vi "Trajectory Builder.vi"() -> ()   [LabVIEW 2018]
uses:
  <vilib>/event_ctls.llb/lveventtype.ctl
panel:
  in  "Time (s)":dbl(slide) scale=0.0..2.3600000000000003 scale format="%#.1g"
  in  "Play":bool
  in  "Destination":u16(ring) items=["Cargo", "Rocket"]
  in  "Direction":u16(ring) items=["Left", "Right", "Other"]
  out "fps":dbl[](graph)
  in  "Limits":T1={"Velocity (fps)"=6.0, "Acceleration (fps^2)"=15.0, "Jerk (fps^3)"=15.0} {"Jerk (fps^3)" min=0.0 step=10.0; "Acceleration (fps^2)" min=0.0; "Velocity (fps)" min=0.0}
  in  "Conditions":T2 {"vFinal (fps)" min=0.0; "vInitial (fps)" min=0.0}
  in  "Append":bool
  in  "Center Flip":bool
  out "WayPoints":cluster{"x":dbl, "y":dbl, "th":dbl}[](array[cluster]) {"th" format="%#_4g"}
  out "Distance (ft)":dbl format="%#.1g"
  in  "Open":i32(listbox)
  out "Path Status":bool
  in  "Sample Period (s)":dbl=0.02
  out "Duration (s)":dbl format="%#.1g"
  in  "Snap to foot":bool
  in  "Angle Limiter":enum16{"90", "45", "15", "1"}(ring)=enum."45"
  in  "Snap robot to baseline":bool
  in  "Filename":string
  in  "Save":bool
  in  "New":bool
  out "Picture":picture
  # "Directions:\nUse mouse to ...\n    move robot position (rectangle with arrow)\n    rotate robot (red arrow)\n    move waypoints (numbered circles)\nClick in open space to add a waypoint\nShift click to delete a waypoint\nHover over a waypoint and use arrow keys to nudge\n\nTime slider and Play button will run robot along path\nto test for collisions\n\nDirection and Destionation are folder selectors for files\n\nNew creates a new path at default location\n\nAppend creates a path"
  # "Trajectory Parameters"
  # "Interaction Options"
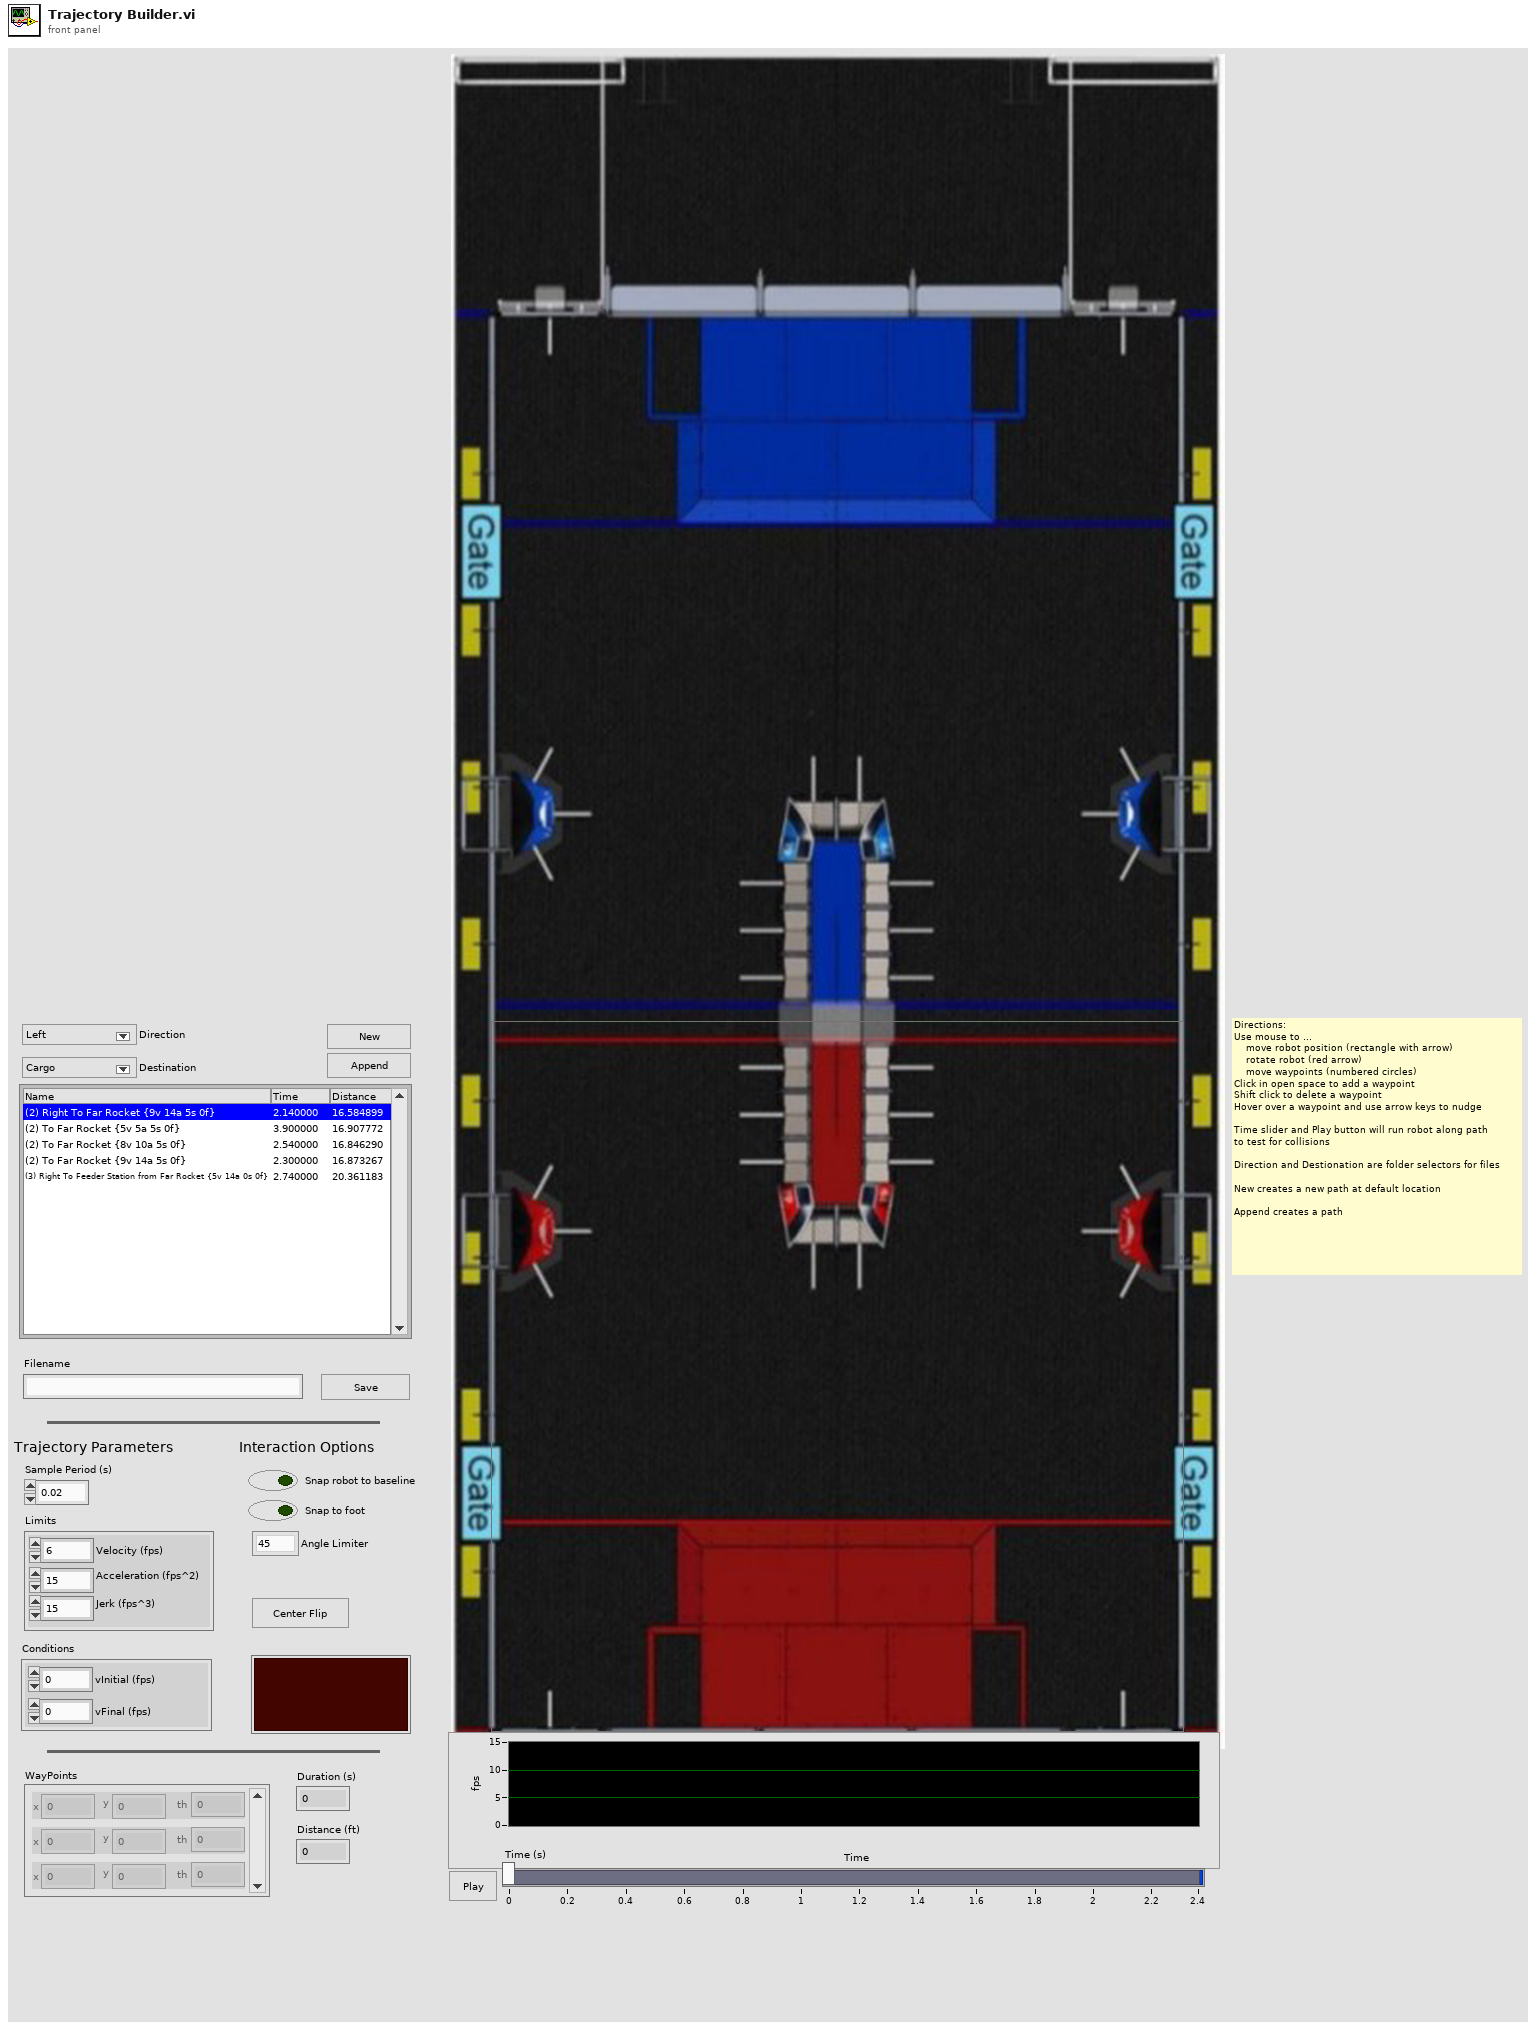
[diagram p1: front panel]
types:
  T1 = cluster{"Velocity (fps)":dbl, "Acceleration (fps^2)":dbl, "Jerk (fps^3)":dbl}
  T2 = cluster{"vInitial (fps)":dbl, "vFinal (fps)":dbl}
  T3 = cluster{"Name":string, "Color":u32, "Style":i32, "Point Style":i32, "Name Visible":bool, "Allow Drag":bool, "Annotation Mode":i32, "Plot":i32, "Index":i32, "Position":cluster{"X":dbl, "Y":dbl}, "X Scale":i32, "Y Scale":u32, "Show Arrow":bool, "Lock Name":bool, "Plot Area":i32, "Label Offset":cluster{"X":dbl, "Y":dbl}}
  T4 = cluster{"Index":i32, "Pt Test Results":enum16{"Miss", "Rect Hit", "Arrow Hit"}}
  T5 = enum16{"Accel Straight", "Const Straight", "Blend", "Circle"}
  T6 = cluster{"Velocity":dbl, "Sample Time":dbl, "Accel":dbl}
  T7 = cluster{"Segment Name":string, "Type":enum16{"Accel Straight", "Const Straight", "Blend", "Circle"}, "Traj Pos Points":cluster{"x":dbl, "y":dbl, "th":dbl}[], "Traj Vel Points":cluster{"V":dbl, "th":dbl}[], "Accel Index":i32, "Decel Index":i32}[]
  T8 = typedef "lveventtype.ctl" = enum32{"Null", "Timeout", "Annotation Menu Selection", "Annotation Menu Selection?", "App Instance Close", "App Instance Close?", "Autoscale Range Change", "Bookmark Info Change", "Cell Edit", "Cell Edit?", "Cursor Grab", "Cursor Grab?", "Cursor Menu Selection", "Cursor Menu Selection?", "Cursor Move", "Cursor Release", "Data Change", "Direction Change", "Display State Change", "Drag Ended", "Drag Enter", "Drag Leave", "Drag Over", "Drag Source Update", "Drag Starting", "Drag Starting?", "Drop", "Exec State Change", "Key Down", "Key Down?", "Key Repeat", "Key Repeat?", "Key Up", "Listbox Double Click", "Menu Activation?", "Menu Selection (App)", "Menu Selection? (App)", "Menu Selection (User)", "Mouse Down", "Mouse Down?", "Mouse Enter", "Mouse Leave", "Mouse Move", "Mouse Up", "Mouse Wheel", "NI Security User Change (App)", "Pane Size", "Panel Close", "Panel Close?", "Panel Resize", "Plot Attribute Change", "Scale Range Change", "Shortcut Menu Activation?", "Shortcut Menu Selection (App)", "Shortcut Menu Selection? (App)", "Shortcut Menu Selection (User)", "Tree Double Click", "Tree Drag", "Tree Drag?", "Tree Drop", "Tree Drop?", "Tree Item Close", "Tree Item Close?", "Tree Item Open", "Tree Item Open?", "User Event", "Value Change"}
  T9 = typedef "LVPoint32TypeDef.ctl" = cluster{"Horizontal":i32, "Vertical":i32}
  T10 = cluster{"Shift":bool, "Ctrl":bool, "Alt":bool, "Cmd":bool, "Opt":bool}
  T11 = typedef "LVPositionTypeDef.ctl" = cluster{"Left":i32, "Top":i32}
  T12 = typedef "LVBoundsTypeDef.ctl" = cluster{"Width":u32, "Height":u32}
  T13 = cluster{"Velocity":dbl, "Accel":dbl, "Accel":dbl}
  T14 = cluster{"Sample Period (s)":dbl, "Limits":cluster{"Velocity (fps)":dbl, "Acceleration (fps^2)":dbl, "Jerk (fps^3)":dbl}, "Conditions":cluster{"vInitial (fps)":dbl, "vFinal (fps)":dbl}}
  T15 = cluster{"Snap robot to baseline":bool, "Snap to foot":bool, "Angle Limiter":enum16{"90", "45", "15", "1"}}
  T16 = cluster{i32, "Pt Test Results":enum16{"Miss", "Rect Hit", "Arrow Hit"}}
  T17 = typedef "eventvkey.ctl" = enum16{"ASCII", "Enter", "Return", "Shift", "Ctrl", "Alt", "Cmd", "Opt", "Caps", "NumLock", "Clear", "Break", "Up", "Down", "Left", "Right", "Insert", "Delete", "Home", "End", "PageUp", "PageDown", "Escape", "Help", "Pause", "ScrollLock", "F1", "F2", "F3", "F4", "F5", "F6", "F7", "F8", "F9", "F10", "F11", "F12", "F13", "F14", "F15", "F16", "F17", "F18", "F19", "F20", "F21", "F22", "F23", "F24", "Play", "VolumeUp", "VolumeDown", "Mute", "Two Byte Char"}
  T18 = cluster{"Horizontal":dbl, "Vertical":dbl, "th":dbl}
  T19 = cluster{"Name":string, "Color":u32, "Style":i32, "Point Style":i32, "Name Visible":bool, "Allow Drag":bool, "Annotation Mode":i32, "Plot":i32, "Index":i32, "Position":cluster{"X":dbl, "Y":dbl}, "X Scale":i32, "Y Scale":u32, "Show Arrow":bool, "Lock Name":bool, "Plot Area":i32, "Label Offset":cluster{"X":dbl, "Y":dbl}}[]
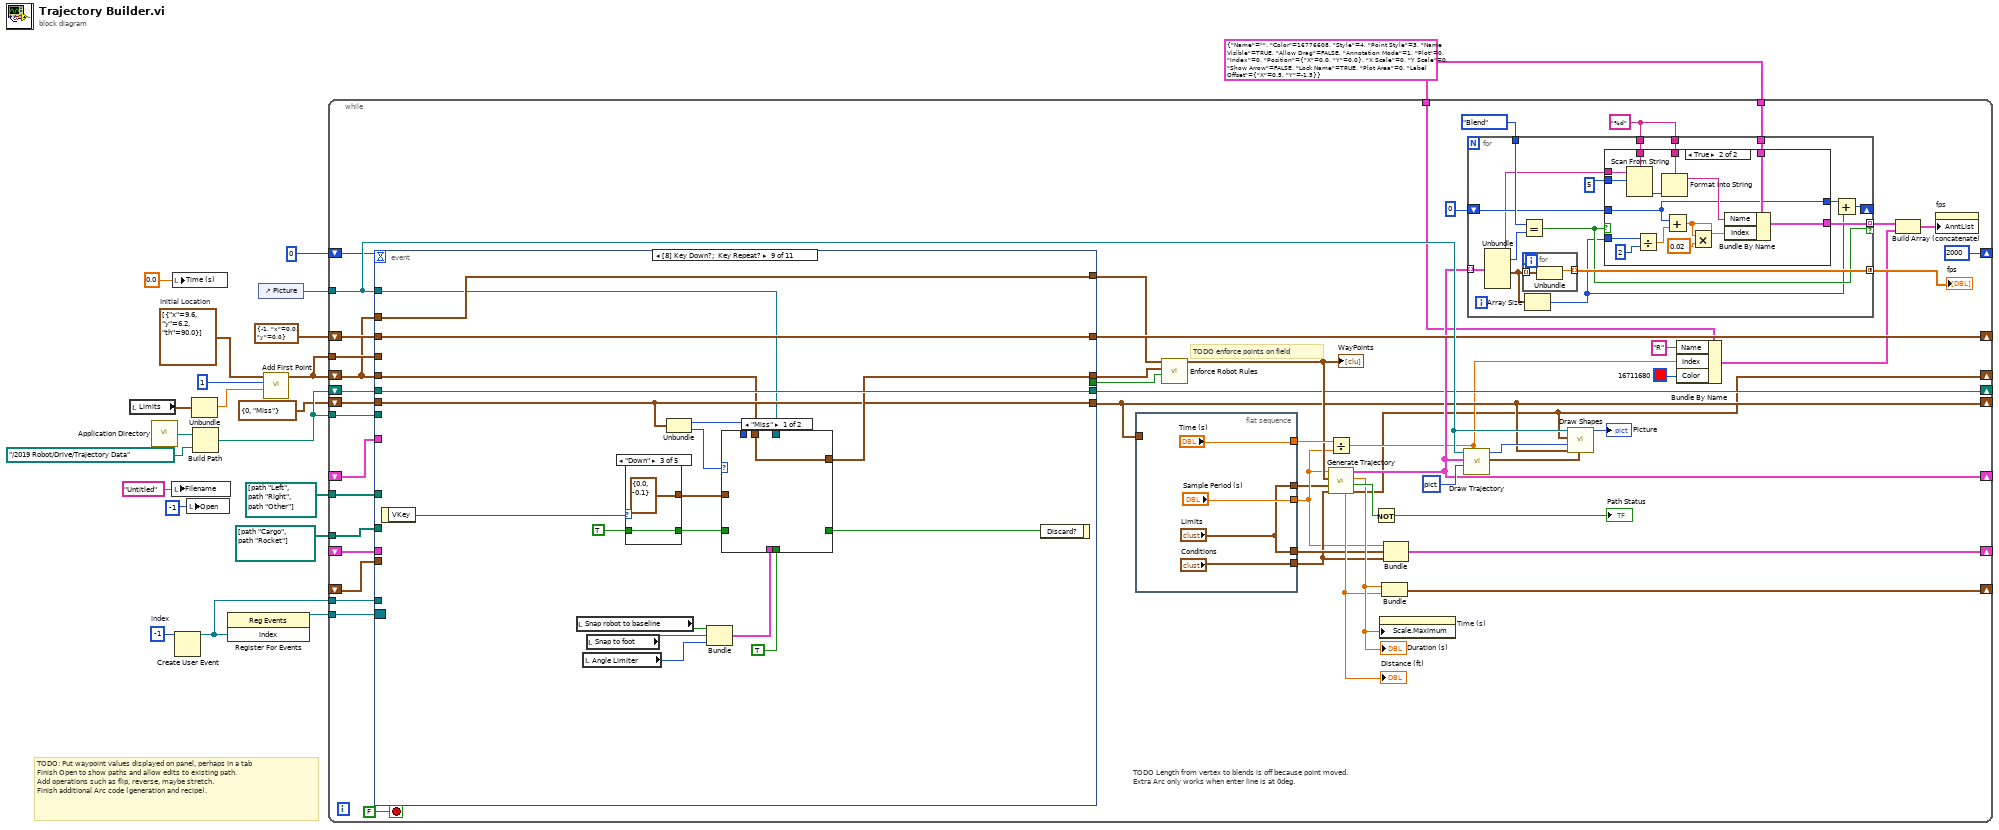
[diagram p0: block diagram]
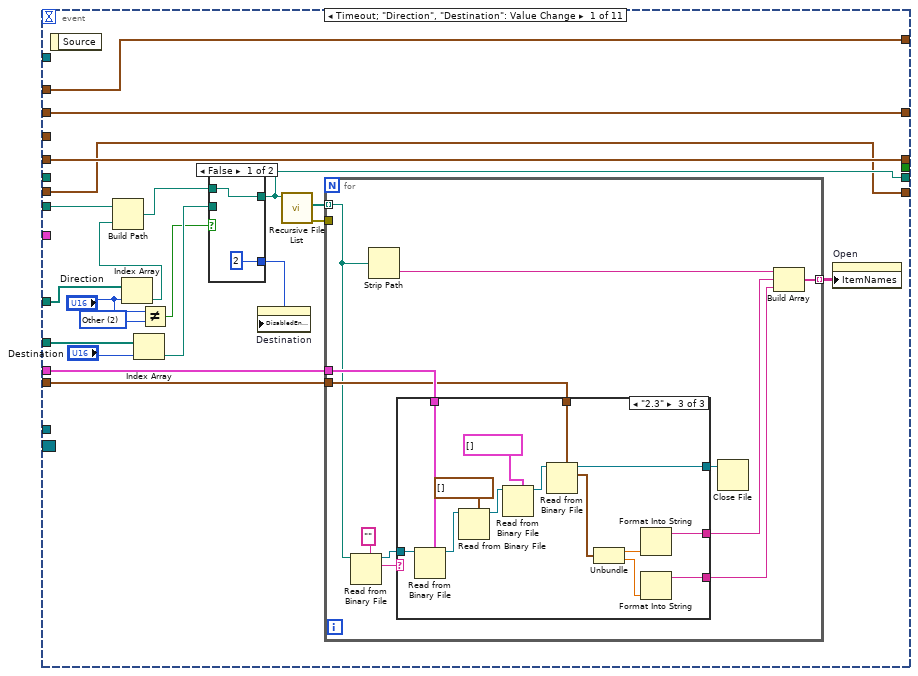
[diagram p3: hidden frame]
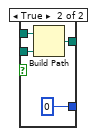
[diagram p4: hidden frame]
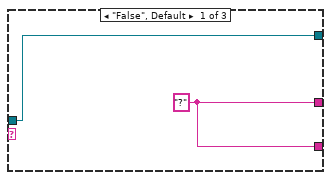
[diagram p5: hidden frame]
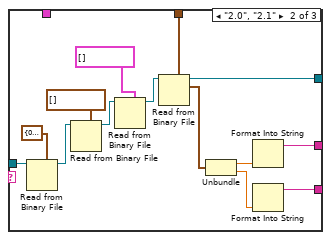
[diagram p6: hidden frame]
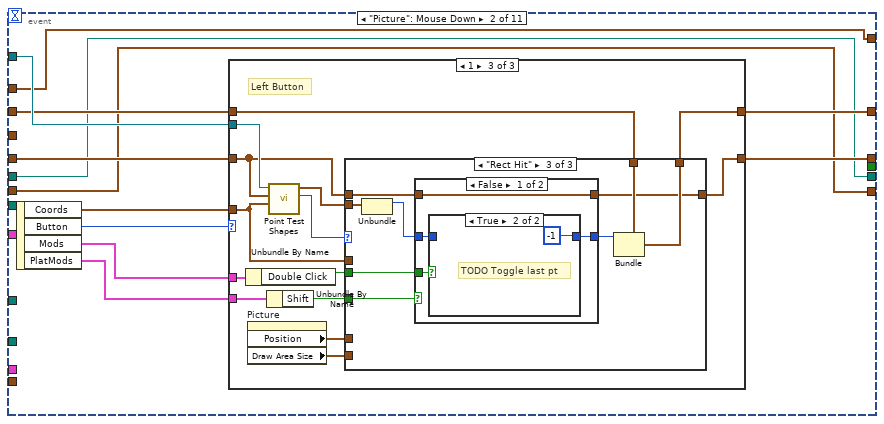
[diagram p7: hidden frame]
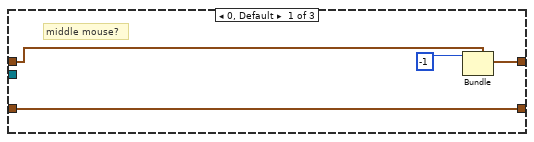
[diagram p8: hidden frame]
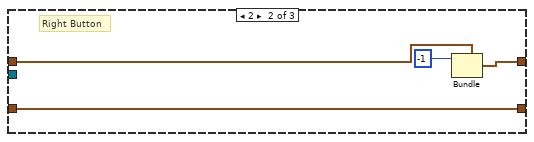
[diagram p9: hidden frame]
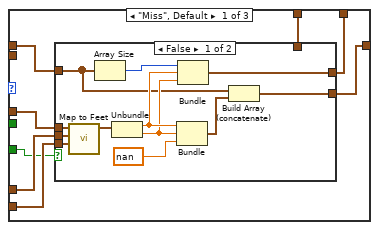
[diagram p10: hidden frame]
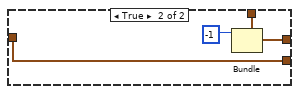
[diagram p11: hidden frame]
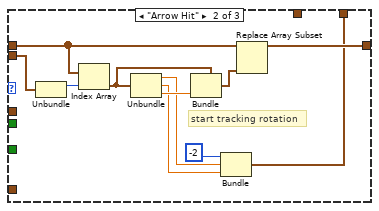
[diagram p12: hidden frame]
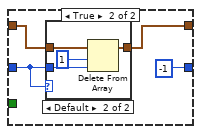
[diagram p14: hidden frame]
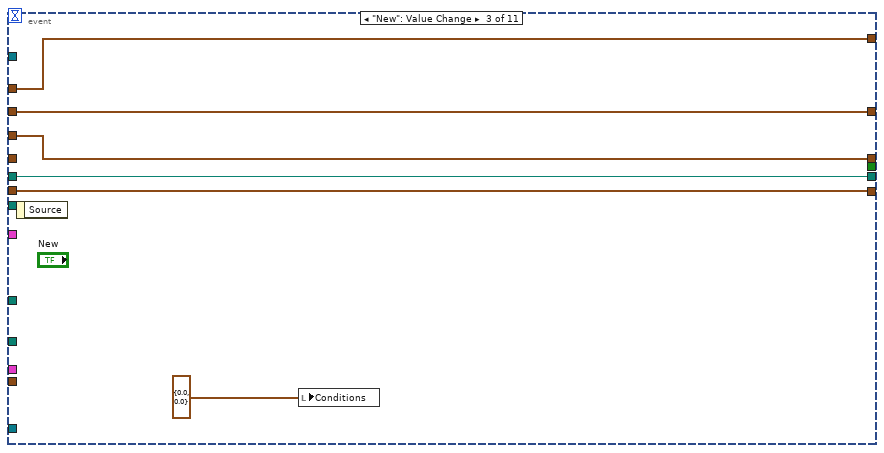
[diagram p16: hidden frame]
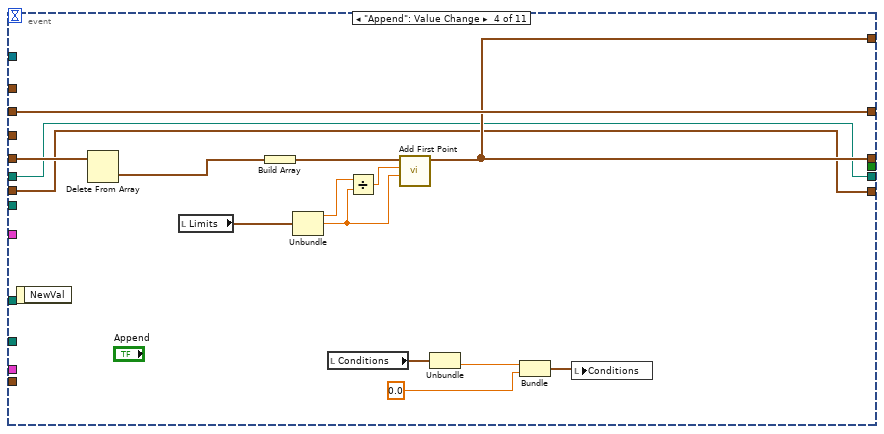
[diagram p17: hidden frame]
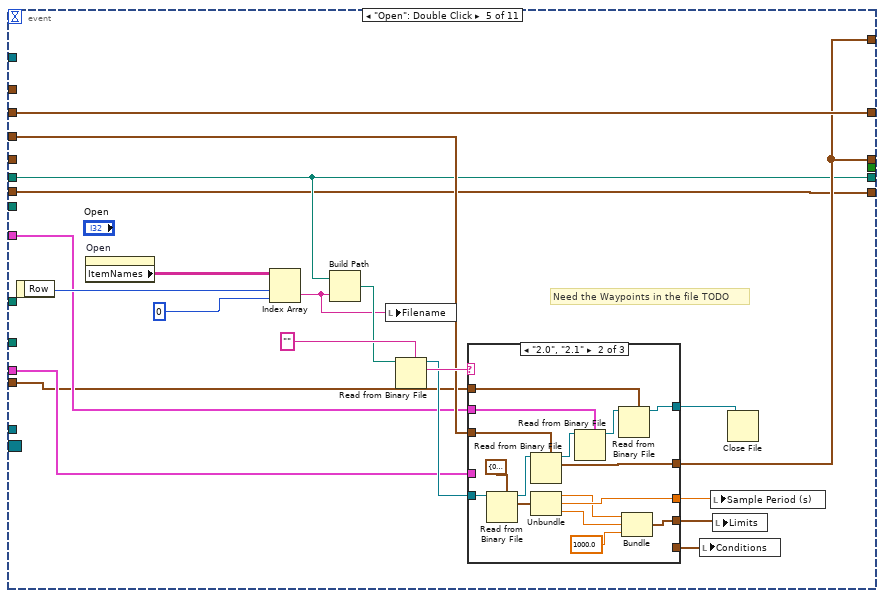
[diagram p18: hidden frame]
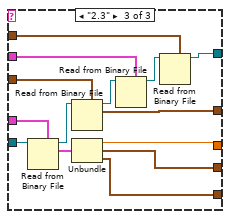
[diagram p20: hidden frame]
diagram:
  w1 = -1  # index
  w4 = T3 {"Name"="", "Color"=16776608, "Style"=4, "Point Style"=3, "Name Visible"=TRUE, "Allow Drag"=FALSE, "Annotation Mode"=1, "Plot"=0, "Index"=0, "Position"={"X"=0.0, "Y"=0.0}, "X Scale"=0, "Y Scale"=0, "Show Arrow"=FALSE, "Lock Name"=TRUE, "Plot Area"=0, "Label Offset"={"X"=0.5, "Y"=-1.5}}
  w18 = cluster{"x":dbl, "y":dbl, "th":dbl}[] [{"x"=9.6, "y"=6.2, "th"=90.0}]  # Initial Location
  # "TODO: Put waypoint values displayed on panel, perhaps in a tab\nFinish Open to show paths and allow edits to existing path.\nAdd operations such as flip, reverse, maybe stretch.\nFinish additional Arc code (generation and recipe)."
  n1 = local read "Limits"() -> (w12:T1)
  n2 = call <vilib>:"Application Directory.vi"() -> ("Application Directory"=w15:path)
  n3 = local write "Filename"("Untitled" ("Filename")) -> ()
  n4 = local write "Time (s)"(0.0 ("Time")) -> ()
  n5 = Create User Event(user event datatype=w1) -> (user event=w2:refnum<user-event>)  [unwired: 1 in, 1 out]
  n6 = local write "Open"(-1) -> ()
  n7 = Unbundle(w12) -> ("Acceleration (fps^2)"=w11:dbl)  [unwired: 2 out]
  n8 = Build Path(base path=w15, name or relative path=path "../2019 Robot/Drive/Trajectory Data") -> (appended path=w8:path)
  n9 = register-events(w2) -> (reference out=w3:refnum<event-registration>)  [unwired: 2 in, 1 out]
  n10 = control-ref of="Picture"() -> (w21:refnum<vi>)
  n11 = call "Add First Point.vi"("Accel (f/s^2)"=w11, "Time (s)"=1 ("th"), "Initial Points"=w18) -> ("Points"=w17:cluster{"x":dbl, "y":dbl, "th":dbl}[])  [unwired: 8 in]
  n12 = while {
    shift-right: [w24] -> _
    shift-left: w17 -> [w60]
    tunnel: w17 -> [w73]
    tunnel: w21 -> [w71]
    shift-right: [w53] -> _
    shift-left: cluster{i32, "x":dbl, "y":dbl} {-1, "x"=0.0, "y"=0.0} ("output cluster") -> [w72]
    shift-right: [w44] -> _
    shift-left: _ -> [w63]
    shift-right: [2000] -> _
    shift-left: 0 -> [w62]
    shift-right: [w59] -> _
    shift-left: _ -> [w58]
    shift-right: [w55] -> _
    shift-left: _ -> [w54]
    tunnel: path[] [path "Left", path "Right", path "Other"] -> [w42]
    tunnel: path[] [path "Cargo", path "Rocket"] -> [w41]
    shift-right: [w39] -> _
    shift-left: w8 -> [w40]
    tunnel: w8 -> [w38]
    shift-right: [w37] -> _
    shift-left: T4 {"Index"=0, "Pt Test Results"=enum."Miss"} ("Results") -> [w36]
    tunnel: w4 -> [w33]
    tunnel: w4 -> [w29]
    tunnel: w3 -> [w23]
    tunnel: w2 -> [w22]
    stop <- FALSE stop-if-true
    w32 = "%d" ("Name")
    # "TODO Length from vertex to blends is off because point moved.\nExtra Arc only works when enter line is at 0deg."
    # "TODO enforce points on field"
    n13 = event shown="[8] Key Down?;  Key Repeat?" {
      selector: w23 -> [_ _ _ _ _ _ _ _ _ _ _]
      dyn-events: _ -> [_ _ _ _ _ _ _ _ _ _ _]
      timeout: w62 -> [_ _ _ _ _ _ _ _ _ _ _]
      tunnel: w60 -> [w132 w188 _ w292 _ w354 w388 w407 w428 w464 w474]
      tunnel: [w132 w187 w278 w290 w301 w355 w388 w408 w436 w464 w474] -> w52
      tunnel: w73 -> [_ _ w278 _ w306 _ _ _ _ _ _]
      tunnel: w71 -> [_ w186 _ _ _ w357 _ _ w434 _ _]
      tunnel: [w112 w180 w273 w279 w294 w356 w385 w401 w435 w460 w472] -> w37
      tunnel: w72 -> [w131 w185 w277 w293 w313 w351 w400 w409 w437 w463 w471]
      tunnel: [w131 w184 w277 w293 w313 w353 w400 w409 w437 w463 w471] -> w53
      tunnel: w63 -> [_ _ _ _ w305 _ w399 _ _ _ _]
      tunnel: w40 -> [_ w181 w274 w280 w295 w345 w386 w402 w439 w462 w473]
      tunnel: [w128 w182 w276 w290 w301 w349 w387 w407 w438 w461 w475] -> w51
      tunnel: w60 -> [w128 w182 w276 _ _ w349 w387 _ w438 w461 w475]
      tunnel: w58 -> [w127 _ _ _ w304 _ w397 _ _ _ _]
      tunnel: w54 -> [w126 _ _ _ w302 _ w393 _ _ _ _]
      tunnel: [_ _ _ _ _ _ _ TRUE ("Flip Over Center") _ _ _] -> w49
      tunnel: w42 -> [w124 _ _ _ _ _ _ _ _ _ _]
      tunnel: w41 -> [w123 _ _ _ _ _ _ _ _ _ _]
      tunnel: [w119 w181 w274 w280 w295 w345 w386 w402 w439 w462 w473] -> w39
      tunnel: w38 -> [w116 _ _ _ _ _ _ _ _ _ _]
      tunnel: w36 -> [w112 w180 w273 w279 w294 _ w385 w401 w435 w460 w472]
      tunnel: w22 -> [_ _ _ _ _ _ _ _ _ w459 w470]
      event Timeout; "Direction", "Destination": Value Change {
        w117 = u16 2 items=["Left", "Right", "Other"] ("Direction")
        n14 = event-data() -> ()  [unwired: 1 in, 1 out]
        n15 = Index Array(array=w124, index="Direction") -> (element=w120:path)
        n16 = Build Path(base path=w116, name or relative path=w120) -> (appended path=w121:path)
        n17 = Index Array(array=w123, index="Destination") -> (element=w115:path)
        n18 = Not Equal?(x="Direction", y=w117) -> (x != y?=w114:bool)
        n19 = case shown="False" w114 {
          tunnel: w121 -> [w134 w138]
          tunnel: [w134 w137] -> w119
          tunnel: w115 -> [_ w136]
          tunnel: [2 0] -> w113
          frame False {
          }
          frame True {
            n20 = Build Path(base path=w138, name or relative path=w136) -> (appended path=w137:path)
          }
        }
        n21 = property on="Destination" class="Ring (strict)"("DisabledEnum"=w113) -> ()  [unwired: 2 in, 2 out]
        n22 = call <vilib>:"Recursive File List.vi"("Folder Path"=w119) -> ("error out"=w125:errorcluster, "All Files in Dir"=w130:path[])  [unwired: 6 in, 3 out]
        n23 = for {
          tunnel: w130 -> [w139] mode=indexing
          tunnel: [w149] -> w129 mode=indexing
          tunnel: w127 -> [w144]
          tunnel: w126 -> [w143]
          tunnel: w125 -> [_]
          n24 = Read from Binary File(5:"", 11:w139) -> (2:w147:string, 3:w146:refnum<file>)  [unwired: 4 in, 2 out]
          n25 = Strip Path(path=w139) -> (name=w140:string)  [unwired: 1 out]
          n26 = case shown="\"2.3\"" w147 {
            tunnel: [w151 w165 w179] -> w142
            tunnel: [w151 w164 w178] -> w141
            tunnel: w146 -> [w150 w163 w177]
            tunnel: [w150 w159 w173] -> w145
            tunnel: w144 -> [_ _ w172]
            tunnel: w143 -> [_ w158 w171]
            frame "False", Default {
              w151 = "?"
            }
            frame "2.0", "2.1" {
              n27 = Read from Binary File(5:T6 {"Velocity"=0.0, "Sample Time"=0.0, "Accel"=0.0}, 11:w163) -> (3:w162:refnum<file>)  [unwired: 4 in, 3 out]
              n28 = Read from Binary File(5:cluster{"x":dbl, "y":dbl, "th":dbl}[] [] ("Points"), 11:w162) -> (3:w161:refnum<file>)  [unwired: 4 in, 3 out]
              n29 = Read from Binary File(5:T7 [] ("Trajectory Data"), 11:w161) -> (3:w160:refnum<file>)  [unwired: 4 in, 3 out]
              n30 = Read from Binary File(5:w158, 11:w160) -> (2:w153:cluster{"Time (s)":dbl, "Distance (ft)":dbl}, 3:w159:refnum<file>)  [unwired: 4 in, 2 out]
              n31 = Unbundle(w153) -> ("Time (s)"=w157:dbl, "Distance (ft)"=w156:dbl)
              n32 = Format Into String(w157) -> (resulting string=w165:string)  [unwired: 3 in, 1 out]
              n33 = Format Into String(w156) -> (resulting string=w164:string)  [unwired: 3 in, 1 out]
            }
            frame "2.3" {
              n34 = Read from Binary File(5:w172, 11:w177) -> (3:w176:refnum<file>)  [unwired: 4 in, 3 out]
              n35 = Read from Binary File(5:cluster{"x":dbl, "y":dbl, "th":dbl}[] [] ("Points"), 11:w176) -> (3:w175:refnum<file>)  [unwired: 4 in, 3 out]
              n36 = Read from Binary File(5:T7 [] ("Trajectory Data"), 11:w175) -> (3:w174:refnum<file>)  [unwired: 4 in, 3 out]
              n37 = Read from Binary File(5:w171, 11:w174) -> (2:w166:cluster{"Time (s)":dbl, "Distance (ft)":dbl}, 3:w173:refnum<file>)  [unwired: 4 in, 2 out]
              n38 = Unbundle(w166) -> ("Time (s)"=w170:dbl, "Distance (ft)"=w169:dbl)
              n39 = Format Into String(w170) -> (resulting string=w179:string)  [unwired: 3 in, 1 out]
              n40 = Format Into String(w169) -> (resulting string=w178:string)  [unwired: 3 in, 1 out]
            }
          }
          n41 = Close File(refnum=w145) -> ()  [unwired: 1 in, 2 out]
          n42 = Build Array(w140, w142, w141) -> (w149:string[])
        }
        n43 = property on="Open" class="MCListbox (strict)"("ItemNames"=w129) -> ()  [unwired: 2 in, 2 out]
      }
      event "Picture": Mouse Down {
        n44 = event-data() -> ("Coords"=w189:T9, "Button"=w191:u16, "Mods"=w190:cluster{"Double Click":bool, "Menu Key":bool}, "PlatMods"=w183:T10)  [unwired: 1 in]
        n45 = case shown="1" w191 {
          tunnel: w190 -> [_ _ w203]
          tunnel: w189 -> [_ _ w208]
          tunnel: w188 -> [w195 w199 w209]
          tunnel: [w195 w199 w213] -> w187
          tunnel: w186 -> [_ _ w210]
          tunnel: w185 -> [w193 w196 w204]
          tunnel: [w192 w198 w205] -> w184
          tunnel: w183 -> [_ _ w201]
          frame 0, Default {
            # "middle mouse?"
            n46 = Bundle(cluster=w193, -1) -> (w192:cluster{i32, "x":dbl, "y":dbl})  [unwired: 2 in]
          }
          frame 2 {
            # "Right Button"
            n47 = Bundle(cluster=w196, -1) -> (w198:cluster{i32, "x":dbl, "y":dbl})  [unwired: 2 in]
          }
          frame 1 {
            # "Left Button"
            n48 = Unbundle By Name(w203) -> ("Double Click"=w202:bool)
            n49 = property on="Picture" class="Pict"() -> ("Position"=w212:T11, "Draw Area Size"=w211:T12)  [unwired: 2 in, 2 out]
            n50 = Unbundle By Name(w201) -> ("Shift"=w200:bool)
            n51 = call "Point Test Shapes.vi"("Coords"=w208, "Points"=w209, "Picture in"=w210) -> ("Pt Test Results"=w207:enum16{"Miss", "Rect Hit", "Arrow Hit"}, "Results"=w206:T4)  [unwired: 7 in]
            n52 = case shown="\"Rect Hit\"" w207 {
              tunnel: w202 -> [_ _ w256]
              tunnel: w209 -> [w217 w245 w250]
              tunnel: w206 -> [_ w243 w257]
              tunnel: [w220 w246 w249] -> w213
              tunnel: w208 -> [w221 _ _]
              tunnel: w212 -> [w219 _ _]
              tunnel: w211 -> [w218 _ _]
              tunnel: [w215 w238 w253] -> w205
              tunnel: w204 -> [w214 _ w254]
              tunnel: w200 -> [w216 _ w251]
              frame "Miss", Default {
                n53 = case shown="False" w216 {
                  tunnel: w221 -> [w233 _]
                  tunnel: [w230 w237] -> w220
                  tunnel: w219 -> [w229 _]
                  tunnel: w218 -> [w228 _]
                  tunnel: w217 -> [w224 w237]
                  tunnel: [w223 w236] -> w215
                  tunnel: w214 -> [_ w234]
                  frame False {
                    n54 = call "Map to Feet.vi"("Draw Area Size"=w228, "Position"=w229, "Coords (px)"=w233) -> ("Point (ft)"=w227:cluster{dbl, dbl})  [unwired: 8 in]
                    n55 = Array Size(array=w224) -> (size(s)=w222:i32)
                    n56 = Unbundle(w227) -> (w226:dbl, w225:dbl)
                    n57 = Bundle(w226, w225, nan) -> (w231:cluster{dbl, dbl, dbl})  [unwired: 1 in]
                    n58 = Bundle(w222, w226, w225) -> (w223:cluster{i32, dbl, dbl})  [unwired: 1 in]
                    n59 = Build Array (concatenate)(w224, w231) -> (w230:cluster{"x":dbl, "y":dbl, "th":dbl}[])
                  }
                  frame True {
                    n60 = Bundle(cluster=w234, -1) -> (w236:cluster{i32, "x":dbl, "y":dbl})  [unwired: 2 in]
                  }
                }
              }
              frame "Arrow Hit" {
                # "start tracking rotation"
                n61 = Unbundle(w243) -> ("Index"=w242:i32)  [unwired: 1 out]
                n62 = Index Array(array=w245, index=w242) -> (element=w244:cluster{"x":dbl, "y":dbl, "th":dbl})
                n63 = Unbundle(w244) -> ("x"=w241:dbl, "y"=w240:dbl, "th"=w248:dbl)
                n64 = Bundle(cluster=w244, "th"=w248) -> (w247:cluster{"x":dbl, "y":dbl, "th":dbl})  [unwired: 2 in]
                n65 = Bundle(-2, "x"=w241, "y"=w240) -> (w238:cluster{i32, "x":dbl, "y":dbl})  [unwired: 1 in]
                n66 = Replace Array Subset(array=w245, new element=w247) -> (w246:cluster{"x":dbl, "y":dbl, "th":dbl}[])  [unwired: 1 in]
              }
              frame "Rect Hit" {
                n67 = Unbundle(w257) -> ("Index"=w255:i32)  [unwired: 1 out]
                n68 = case shown="False" w251 {
                  tunnel: w256 -> [w261 _]
                  tunnel: w255 -> [w260 w264]
                  tunnel: [w259 -1 ("length")] -> w252
                  tunnel: w250 -> [w258 w267]
                  tunnel: [w258 w266] -> w249
                  frame False {
                    n69 = case shown="True" w261 {
                      tunnel: w260 -> [w262 _]
                      tunnel: [w262 -1] -> w259
                      frame False {
                      }
                      frame True {
                        # "TODO Toggle last pt"
                      }
                    }
                  }
                  frame True {
                    n70 = case shown="Default" w264 {
                      tunnel: w267 -> [w268 w272]
                      tunnel: w264 -> [_ w271]
                      tunnel: [w268 w269] -> w266
                      frame 0 {
                      }
                      frame Default {
                        n71 = Delete From Array(array=w272, length=1, index=w271) -> (array with subset deleted=w269:cluster{"x":dbl, "y":dbl, "th":dbl}[])  [unwired: 1 out]
                      }
                    }
                  }
                }
                n72 = Bundle(cluster=w254, w252) -> (w253:cluster{i32, "x":dbl, "y":dbl})  [unwired: 2 in]
              }
            }
          }
        }
      }
      event "New": Value Change {
        n73 = event-data() -> ()  [unwired: 1 in, 1 out]
        n74 = local write "Conditions"(T2 {"vInitial (fps)"=0.0, "vFinal (fps)"=0.0} ("Conditions")) -> ()
      }
      event "Append": Value Change {
        n75 = event-data() -> ()  [unwired: 1 in, 1 out]
        n76 = Delete From Array(array=w292) -> (deleted portion=w289:cluster{"x":dbl, "y":dbl, "th":dbl})  [unwired: 2 in, 1 out]
        n77 = local read "Limits"() -> (w283:T1)
        n78 = Build Array(w289) -> (w288:cluster{"x":dbl, "y":dbl, "th":dbl}[])
        n79 = Unbundle(w283) -> ("Velocity (fps)"=w282:dbl, "Acceleration (fps^2)"=w281:dbl)  [unwired: 1 out]
        n80 = local read "Conditions"() -> (w287:T2)
        n81 = Divide(x=w282, y=w281) -> (x/y=w291:dbl)
        n82 = call "Add First Point.vi"("Accel (f/s^2)"=w281, "Time (s)"=w291, "Initial Points"=w288) -> ("Points"=w290:cluster{"x":dbl, "y":dbl, "th":dbl}[])  [unwired: 8 in]
        n83 = Unbundle(w287) -> ("vFinal (fps)"=w286:dbl)  [unwired: 1 out]
        n84 = Bundle("vFinal (fps)"=w286, 0.0) -> (w285:cluster{"vFinal (fps)":dbl, dbl})  [unwired: 1 in]
        n85 = local write "Conditions"(w285) -> ()
      }
      event "Open": Double Click {
        # "Need the Waypoints in the file TODO"
        n86 = event-data() -> ("Row"=w311:i32)  [unwired: 1 in]
        n87 = property on="Open" class="MCListbox (strict)"() -> ("ItemNames"=w312:string[][])  [unwired: 2 in, 2 out]
        n88 = Index Array(array=w312, index (row)=w311, index (col)=0 ("disabled index (col)")) -> (element=w299:string)
        n89 = Build Path(base path=w295, name or relative path=w299) -> (appended path=w300:path)
        n90 = local write "Filename"(w299) -> ()
        n91 = Read from Binary File(5:"", 11:w300) -> (2:w308:string, 3:w307:refnum<file>)  [unwired: 4 in, 2 out]
        n92 = case shown="\"2.0\", \"2.1\"" w308 {
          tunnel: w307 -> [w314 w329 w343]
          tunnel: w304 -> [_ _ w332]
          tunnel: w306 -> [_ w327 w341]
          tunnel: [_ w326 w340] -> w301
          tunnel: w305 -> [_ w325 w339]
          tunnel: w302 -> [_ w323 w337]
          tunnel: [w314 w321 w335] -> w303
          tunnel: [_ w319 w334] -> w298
          tunnel: [_ w318 w333] -> w297
          tunnel: [_ _ w331] -> w296
          frame "False", Default {
          }
          frame "2.0", "2.1" {
            n93 = Read from Binary File(5:T6 {"Velocity"=0.0, "Sample Time"=0.0, "Accel"=0.0}, 11:w329) -> (2:w330:T6, 3:w328:refnum<file>)  [unwired: 4 in, 2 out]
            n94 = Read from Binary File(5:w327, 11:w328) -> (2:w326:cluster{"x":dbl, "y":dbl, "th":dbl}[], 3:w324:refnum<file>)  [unwired: 4 in, 2 out]
            n95 = Unbundle(w330) -> ("Velocity"=w317:dbl, "Sample Time"=w319:dbl, "Accel"=w316:dbl)
            n96 = Read from Binary File(5:w325, 11:w324) -> (3:w322:refnum<file>)  [unwired: 4 in, 3 out]
            n97 = Read from Binary File(5:w323, 11:w322) -> (3:w321:refnum<file>)  [unwired: 4 in, 3 out]
            n98 = Bundle("Velocity"=w317, "Accel"=w316, "Accel"=1000.0) -> (w318:T13)  [unwired: 1 in]
          }
          frame "2.3" {
            n99 = Read from Binary File(5:w332, 11:w343) -> (2:w344:T14, 3:w342:refnum<file>)  [unwired: 4 in, 2 out]
            n100 = Read from Binary File(5:w341, 11:w342) -> (2:w340:cluster{"x":dbl, "y":dbl, "th":dbl}[], 3:w338:refnum<file>)  [unwired: 4 in, 2 out]
            n101 = Unbundle(w344) -> ("Sample Period (s)"=w334:dbl, "Limits"=w333:T1, "Conditions"=w331:T2)
            n102 = Read from Binary File(5:w339, 11:w338) -> (3:w336:refnum<file>)  [unwired: 4 in, 3 out]
            n103 = Read from Binary File(5:w337, 11:w336) -> (3:w335:refnum<file>)  [unwired: 4 in, 3 out]
          }
        }
        n104 = local write "Conditions"(w296) -> ()
        n105 = local write "Sample Period (s)"(w298) -> ()
        n106 = local write "Limits"(w297) -> ()
        n107 = Close File(refnum=w303) -> ()  [unwired: 1 in, 2 out]
      }
      event "Picture": Mouse Move; "Picture": Mouse Up {
        n108 = event-data() -> ("Type"=w352:T8, "Coords"=w358:T9)  [unwired: 1 in]
        n109 = Unbundle(w351) -> (w350:i32)  [unwired: 2 out]
        n110 = case shown="-1" w350 {
          selector: w350 -> [w368 _]
          tunnel: w358 -> [w377 w384]
          tunnel: w357 -> [w363 w383]
          tunnel: [w375 w382] -> w356
          tunnel: [w372 w381] -> w355
          tunnel: w354 -> [w373 w381]
          tunnel: [w369 w380] -> w353
          tunnel: w351 -> [w359 w380]
          tunnel: w352 -> [w370 _]
          tunnel: "Snap to foot" -> [w365 _]
          tunnel: "Snap robot to baseline" -> [w366 _]
          tunnel: "Angle Limiter" -> [w367 _]
          frame Default {
            # "Mouse up changes indes to break tracking,\notherwise update coords"
            n111 = property on="Picture" class="Pict"() -> ("Position"=w378:T11, "Draw Area Size"=w379:T12)  [unwired: 2 in, 2 out]
            n112 = Bundle("Snap robot to baseline"=w366, "Snap to foot"=w365, "Angle Limiter"=w367) -> (w364:T15)  [unwired: 1 in]
            n113 = call "Map to Feet.vi"("Draw Area Size"=w379, "Position"=w378, "Coords (px)"=w377) -> ("Point (ft)"=w376:cluster{dbl, dbl})  [unwired: 8 in]
            n114 = Equal?(x=lveventtype."Mouse Up" ("Type"), y=w370) -> (x = y?=w362:bool)
            n115 = call "Handle Pos and Rot.vi"("Mouse Up"=w362, "Picture in"=w363, "Option"=w364, "Coord (ft)"=w376, "Index"=w368, "Points in"=w373) -> ("Points out"=w372:cluster{"x":dbl, "y":dbl, "th":dbl}[])  [unwired: 5 in]
            n116 = Bundle(cluster=w359, -1) -> (w360:cluster{i32, "x":dbl, "y":dbl})  [unwired: 2 in]
            n117 = Bundle(w368, "Pt Test Results"=enum16{"Miss", "Rect Hit", "Arrow Hit"}."Rect Hit") -> (w375:T16)  [unwired: 1 in]
            n118 = Select(t=w360, s=w362, f=w359) -> (s? t:f=w369:cluster{i32, "x":dbl, "y":dbl})
          }
          frame -1 {
            n119 = call "Point Test Shapes.vi"("Coords"=w384, "Points"=w381, "Picture in"=w383) -> ("Results"=w382:T4)  [unwired: 7 in, 1 out]
          }
        }
      }
      event "Save": Value Change {
        n120 = event-data() -> ()  [unwired: 1 in, 1 out]
        n121 = Build Path(base path=w386, name or relative path="Filename") -> (appended path=w391:path)
        n122 = Write to Binary File(file (use dialog)=w391, data="2.3") -> (refnum out=w390:refnum<file>)  [unwired: 4 in, 2 out]
        n123 = Write to Binary File(file (use dialog)=w390, data=w397) -> (refnum out=w396:refnum<file>)  [unwired: 4 in, 2 out]
        n124 = Write to Binary File(file (use dialog)=w396, data=w387) -> (refnum out=w395:refnum<file>)  [unwired: 4 in, 2 out]
        n125 = Write to Binary File(file (use dialog)=w395, data=w399) -> (refnum out=w394:refnum<file>)  [unwired: 4 in, 2 out]
        n126 = Write to Binary File(file (use dialog)=w394, data=w393) -> (refnum out=w392:refnum<file>)  [unwired: 4 in, 2 out]
        n127 = Close File(refnum=w392) -> ()  [unwired: 1 in, 2 out]
      }
      event "Time (s)", "Snap to foot", "Angle Limiter", "Snap robot to baseline", "Limits", "Sample Period (s)", "Center Flip", "Conditions": Value Change {
        # "Changes to any of these control will run the diagram to update the preview"
        n128 = event-data() -> ("CtlRef"=w405:refnum<vi>)  [unwired: 1 in]
        n129 = control-ref of="Center Flip"() -> (w406:refnum<vi>)
        n130 = Equal?(x=w406, y=w405) -> (x = y?=w404:bool)
        n131 = case shown="True" w404 {
          tunnel: w407 -> [w410 w412]
          tunnel: [w410 w411] -> w408
          frame False {
          }
          frame True {
            n132 = for {
              tunnel: w412 -> [w420] mode=indexing
              tunnel: [w413] -> w411 mode=indexing
              n133 = Unbundle(w420) -> ("x"=w419:dbl, "y"=w415:dbl, "th"=w414:dbl)
              n134 = Negate(x=w419) -> (-x=w418:dbl)
              n135 = Add(x=27.0 ("y"), y=w418) -> (x+y=w416:dbl)
              n136 = Bundle(w416, "y"=w415, "th"=w414) -> (w413:cluster{dbl, "y":dbl, "th":dbl})  [unwired: 1 in]
            }
          }
        }
      }
      event Key Down?; event type 5.0.x8000000b {
        n137 = event-data() -> ("VKey"=w424:T17)  [unwired: 1 in]
        n138 = local read "Snap robot to baseline"() -> (w433:bool)
        n139 = local read "Angle Limiter"() -> (w431:enum16{"90", "45", "15", "1"})
        n140 = local read "Snap to foot"() -> (w432:bool)
        n141 = case shown="\"Down\"" w424 {
          tunnel: [cluster{dbl, dbl} {0.0, 0.0} ("Coord (ft)") cluster{dbl, dbl} {0.0, 0.1} ("Coord (ft)") cluster{dbl, dbl} {0.0, -0.1} ("Coord (ft)") cluster{dbl, dbl} {-0.1, 0.0} ("Coord (ft)") cluster{dbl, dbl} {0.1, 0.0} ("Coord (ft)")] -> w426
          tunnel: [_ w450 w452 w454 w456] -> w422
          tunnel: TRUE ("Delta") -> [_ w450 w452 w454 w456]
          frame Default {
          }
          frame "Up" {
          }
          frame "Down" {
          }
          frame "Left" {
          }
          frame "Right" {
          }
        }
        n142 = Unbundle(w435) -> ("Index"=w429:i32, "Pt Test Results"=w423:enum16{"Miss", "Rect Hit", "Arrow Hit"})
        n143 = Bundle("Snap robot to baseline"=w433, "Snap to foot"=w432, "Angle Limiter"=w431) -> (w430:T15)  [unwired: 1 in]
        n144 = case shown="\"Miss\"" w423 {
          tunnel: [w440 w448] -> w436
          tunnel: w434 -> [_ w447]
          tunnel: w430 -> [_ w446]
          tunnel: w429 -> [_ w445]
          tunnel: w428 -> [w440 w444]
          tunnel: TRUE ("Delta") -> [_ w443]
          tunnel: w426 -> [_ w442]
          tunnel: w422 -> [_ w441]
          tunnel: [_ w441] -> w421
          frame "Miss" {
          }
          frame "Rect Hit", Default {
            n145 = call "Handle Pos and Rot.vi"("Delta"=w443, "Picture in"=w447, "Option"=w446, "Coord (ft)"=w442, "Index"=w445, "Points in"=w444) -> ("Points out"=w448:cluster{"x":dbl, "y":dbl, "th":dbl}[])  [unwired: 5 in]
          }
        }
        n146 = event-data("Discard?"=w421) -> ()  [unwired: 1 in, 1 out]
      }
      event "Play": Value Change {
        n147 = event-data() -> ()  [unwired: 1 in, 1 out]
        n148 = Generate User Event(user event=w459, event data cluster=0 ("event data")) -> ()  [unwired: 2 in, 2 out]
      }
      event User Event {
        n149 = event-data() -> ("index"=w469:i32)  [unwired: 1 in]
        n150 = local read "Duration (s)"() -> (w466:dbl)
        n151 = Multiply(x=w469, y=0.02) -> (x*y=w465:dbl)
        n152 = Less Or Equal?(x=w465, y=w466) -> (x <= y?=w468:bool)
        n153 = case shown="True" w468 {
          tunnel: w470 -> [_ w479]
          tunnel: w469 -> [_ w477]
          tunnel: w465 -> [_ w476]
          frame False {
          }
          frame True {
            n154 = Increment(x=w477) -> (x+1=w478:i32)
            n155 = local write "Time (s)"(w476) -> ()
            n156 = Generate User Event(user event=w479, event data cluster=w478) -> ()  [unwired: 2 in, 2 out]
          }
        }
      }
    }
    n157 = flat-sequence {
      tunnel: ["Time (s)"] -> w68
      tunnel: ["Sample Period (s)"] -> w46
      tunnel: w37 -> [_]
      tunnel: ["Conditions"] -> w47
      tunnel: ["Limits"] -> w48
      tunnel: ["Limits"] -> w45
      frame #0 {
      }
    }
    n158 = call "Enforce Robot Rules.vi"("Disable"=w49, "New Points"=w52, "Original Points"=w51) -> ("Points out"=w50:cluster{"x":dbl, "y":dbl, "th":dbl}[])  [unwired: 8 in]
    "WayPoints" <- w50
    n159 = Divide(x=w68, y=w46) -> (x/y=w31:dbl)
    n160 = call "Generate Trajectory.vi"("Conditions"=w47, "Limits"=w45, "WayPoints"=w50, "Sample Period (s)"=w46) -> ("Updated Waypoints"=w24:cluster{"x":dbl, "y":dbl, "th":dbl}[], "Valid"=w65:bool, "Time (s)"=w57:dbl, "Trajectory Data"=w44:T7, "Distance (ft)"=w56:dbl)  [unwired: 3 in]
    "Duration (s)" <- w57
    "Distance (ft)" <- w56
    n161 = Not(x=w65) -> (.not. x?=→"Path Status":bool)
    n162 = property on="Time (s)" class="Slide (strict)"("Scale.Maximum"=w57) -> ()  [unwired: 2 in, 2 out]
    n163 = Bundle("Time (s)"=w57, "Distance (ft)"=w56) -> (w55:cluster{"Time (s)":dbl, "Distance (ft)":dbl})  [unwired: 1 in]
    n164 = Bundle("Sample Period (s)"=w46, "Limits"=w48, "Conditions"=w47) -> (w59:T14)  [unwired: 1 in]
    n165 = call "Draw Trajectory.vi"("Robot Index"=w31, "new picture in"=picture data[5B] ("new picture"), "Trajectory Data"=w44, "Picture in"=w71) -> ("Output Point"=w67:T18, "new picture"=w69:picture)  [unwired: 6 in]
    n166 = for {
      tunnel: w44 -> [w90] mode=indexing
      tunnel: [w89] -> w43 mode=concatenating
      tunnel: T5."Blend" ("Type") -> [w88]
      shift-right: [w77] -> _
      shift-left: 0 -> [w85]
      tunnel: [w80] -> w26 mode=indexing if=w79
      tunnel: w33 -> [w84]
      tunnel: w32 -> [w82]
      tunnel: w32 -> [w81]
      n167 = Unbundle(w90) -> ("Segment Name"=w83:string, "Type"=w87:T5, "Traj Vel Points"=w86:cluster{"V":dbl, "th":dbl}[])  [unwired: 3 out]
      n168 = Equal?(x=w88, y=w87) -> (x = y?=w79:bool)
      n169 = for {
        tunnel: w86 -> [w107] mode=indexing
        tunnel: [w106] -> w89 mode=indexing
        n170 = Unbundle(w107) -> ("V"=w106:dbl)  [unwired: 1 out]
      }
      n171 = Array Size(array=w86) -> (size(s)=w76:i32)
      n172 = case shown="True" w79 {
        tunnel: w85 -> [w91 w96]
        tunnel: [w91 w96] -> w78
        tunnel: w84 -> [_ w104]
        tunnel: w83 -> [_ w103]
        tunnel: w82 -> [_ w102]
        tunnel: w81 -> [_ w101]
        tunnel: [_ w98] -> w80
        tunnel: w76 -> [_ w93]
        tunnel: 5 -> [_ w92]
        frame False {
        }
        frame True {
          n173 = Scan From String(format string=w102, input string=w103, initial scan location=w92) -> (output 1=w100:i32)  [unwired: 2 in, 3 out]
          n174 = Divide(x=w93, y=2) -> (x/y=w94:dbl)
          n175 = Format Into String(format string=w101, w100) -> (resulting string=w99:string)  [unwired: 2 in, 1 out]
          n176 = Add(x=w96, y=w94) -> (x+y=w97:dbl)
          n177 = Multiply(x=w97, y=0.02) -> ()  [unwired: 1 out]
          n178 = Bundle By Name(cluster=w104, "Name"=w99, "Index"=w97) -> (w98:T3)
        }
      }
      n179 = Add(x=w78, y=w76) -> (x+y=w77:i32)
    }
    "fps" <- w43
    n180 = call "Draw Shapes.vi"("Output Point"=w67, "Results"=w37, "new picture in"=w69, "Points"=w24, "Picture in"=w71) -> ("new picture out"=→"Picture":picture)  [unwired: 6 in]
    n181 = Bundle By Name(cluster=w29, "Name"="R", "Index"=w31, "Color"=u32 16711680) -> (w27:T3)
    n182 = Build Array (concatenate)(w26, w27) -> (w25:T19)
    n183 = property on="fps" class="WFGraph (strict)"("AnntList"=w25) -> ()  [unwired: 2 in, 2 out]
  }
